vi "TDMS_Ctrl.vi"(0 "Create TDMS?":refnum<vi>, 1 "Data":dbl[][](array[numeric]), 2 "Filename.TDMS":path=path "Vaisala Data.tdms", 3 "group name":string="myRIO Data", 4 "Title":string="IOT Project", 5 "error in (no error)":errorcluster) -> (14 "file path out":path, 19 "error out":errorcluster)   [LabVIEW 2015]
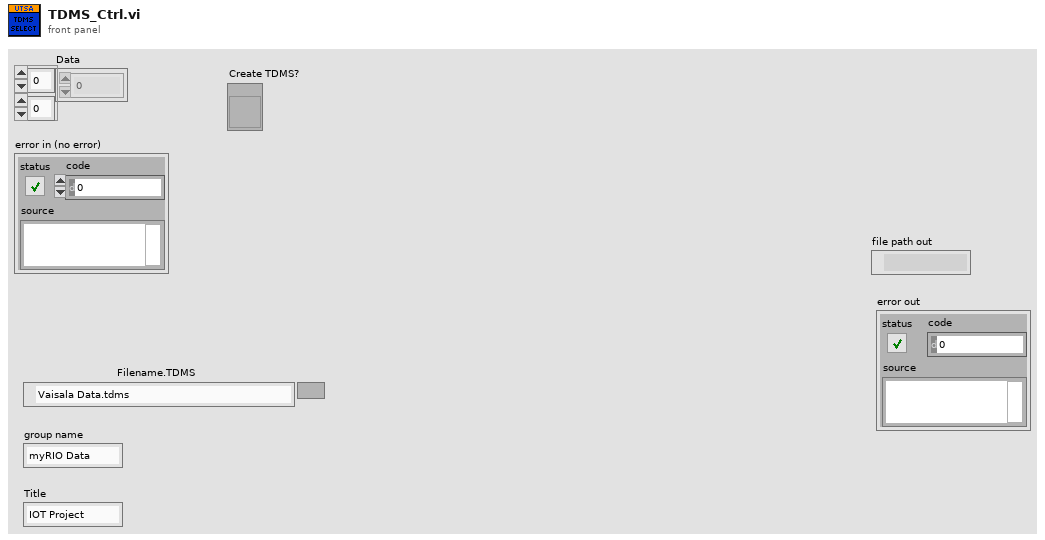
[diagram p1: front panel]
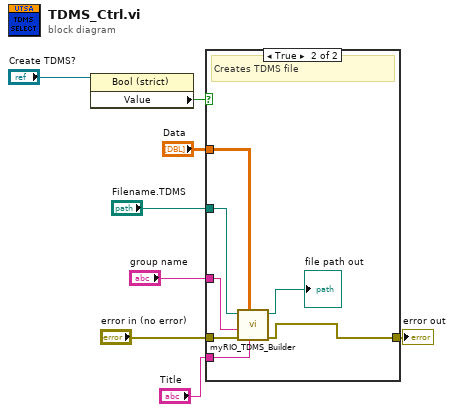
[diagram p0: block diagram]
diagram:
  n1 = property class="Bool (strict)"(reference="Create TDMS?") -> ("Value"=w4:bool)  [unwired: 1 in, 2 out]
  n2 = case shown="True" w4 {
    tunnel: "Data" -> [_ w16]
    tunnel: "error in (no error)" -> [w9 w15]
    tunnel: [w9 w11] -> w8
    tunnel: "Title" -> [_ w14]
    tunnel: "group name" -> [_ w13]
    tunnel: "Filename.TDMS" -> [_ w12]
    frame False {
    }
    frame True {
      # "Creates TDMS file"
      n3 = call "myRIO_TDMS_Builder.vi"("Title"=w14, "Data"=w16, "error in (no error)"=w15, "group name"=w13, "Filename.TDMS"=w12) -> ("error out"=w11:errorcluster, "file path out"=→"file path out":path)  [unwired: 5 in]
    }
  }
  "error out" <- w8
